vi "clean.vi"(8 "Error In":errorcluster, 10 "Sim/Live":bool, 11 "SystemID":i32) -> (0 "Error Out":errorcluster)   [LabVIEW 2019]
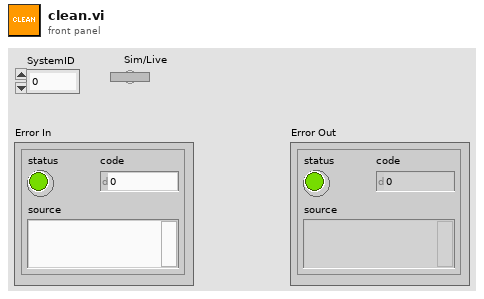
[diagram p1: front panel]
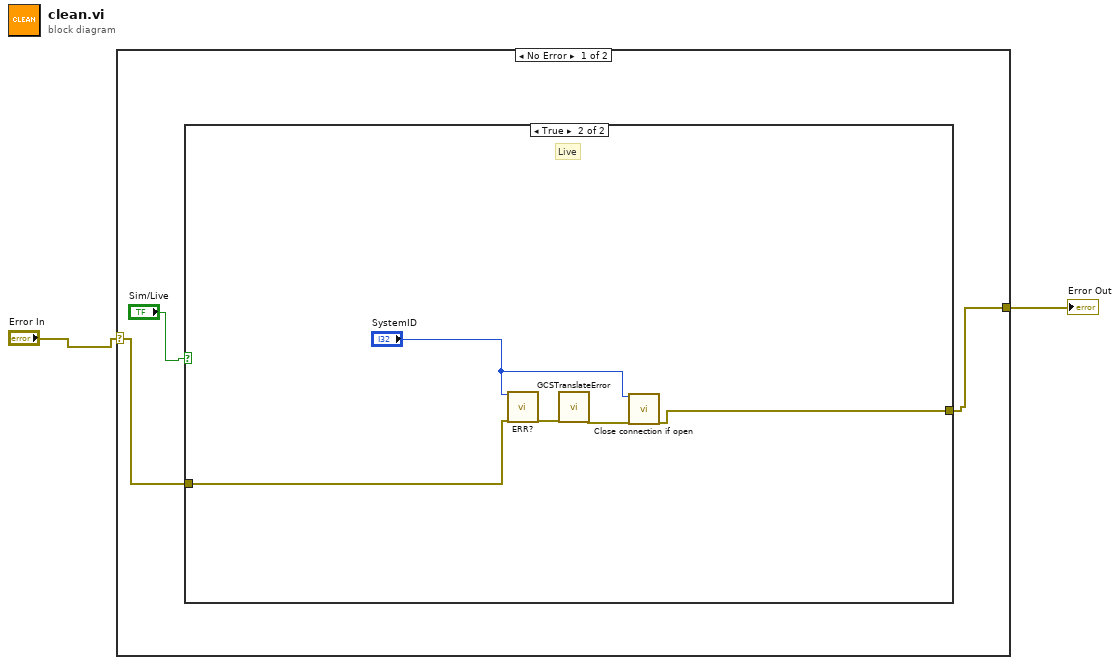
[diagram p0: block diagram]
diagram:
  n1 = case shown="No Error" "Error In" {
    selector: "Error In" -> [w5 w12]
    tunnel: [w4 w12] -> w1
    frame No Error {
      n2 = case shown="True" "Sim/Live" {
        tunnel: w5 -> [w6 w7]
        tunnel: [w6 w9] -> w4
        frame False {
          # "Sim"
        }
        frame True {
          # "Live"
          n3 = call "ERR?.vi"("System no."="SystemID", "error in"=w7) -> ("error out"=w11:errorcluster)  [unwired: 17 out]
          n4 = call "GCSTranslateError.vi"("error in"=w11) -> ("error out"=w10:errorcluster)  [unwired: 18 out]
          n5 = call "Close connection if open.vi"("System no."="SystemID", "error in"=w10) -> ("error out"=w9:errorcluster)  [unwired: 1 in, 16 out]
        }
      }
    }
    frame Error {
    }
  }
  "Error Out" <- w1
